vi "APU + 1 Data Replay.vi"() -> ()   [LabVIEW 2013]
uses:
  IP Source/APU/Settings.ctl
  IP Source/APU/Output.ctl
  IP Source/APU/Input.ctl
  IP Source/Analog Replay/Settings.ctl
  IP Source/Analog Replay/Input.ctl
  IP Source/Analog Replay/Load Input.ctl
  IP Source/Version Token.ctl
  IP Source/APU/Shared Settings.ctl
  <vilib>/Platform/TimedLoop/XDataNode/timing_clust.ctl
  <vilib>/Platform/TimedLoop/XDataNode/nitl_modes.ctl
  <vilib>/Platform/TimedLoop/XDataNode/wakeup.ctl
  <vilib>/rvi/DataTransferAndStorage/Container/Common/niFpgaContainerGetUniqueNameForEmu.vi
  <vilib>/rvi/DataTransferAndStorage/Container/Common/niFpgaContainerSetEmuInfo.vi
  <vilib>/rvi/eio/common/nirviEmuReportErrorAndStop.vi
  <vilib>/rvi/Emulation/niFpgaSctlEmulationGetInTimedLoop.vi
  <vilib>/rvi/Emulation/niFpgaEmulationReportErrorSimple.vi
  <vilib>/rvi/Emulation/niFpgaGetClockAttributes.vi
  <vilib>/rvi/Emulation/niFpgaCriticalErrorInLSC.vi
  <vilib>/rvi/eio/common/nirviEmuTemplateMethod_errors.vi
  <vilib>/Platform/TimedLoop/XDataNode/XDataNode.xnode
  <vilib>/rvi/LocalResourceManager/LocalResourceManager.xnode
  <vilib>/eio/EIONode/EIONode.xnode
  <vilib>/Platform/TimedLoop/XDataNode/XDNodeRunTimeDep.lvlib
  IP Source/APU/APU.lvlib
  IP Source/Analog Replay/Analog Replay.lvlib
  IP Source/Engine Simulation Toolkit.lvlib
panel:
  in  "go.my apu":bool
  in  "shared settings.my apu":T1 {"cycle start" format="%#.15g"}
  in  "est.version":T2
  in  "load input.my replay":T3={"Data"=[0, 0, 0, 0, 0, 0, 0, 0, 0, 0, 0, 0, 0, 0, 0, 0], "LoadOffset"=0, "Done"=FALSE}
  in  "input.my replay":T4 caption="input"
  in  "settings.my replay":T5 caption="settings"
  in  "input.my apu":T6={"desired speed"=0.0, "reset"=TRUE} caption="input"
  out "output.my apu":T7 caption="output"
  in  "settings.my apu":T8 caption="settings"
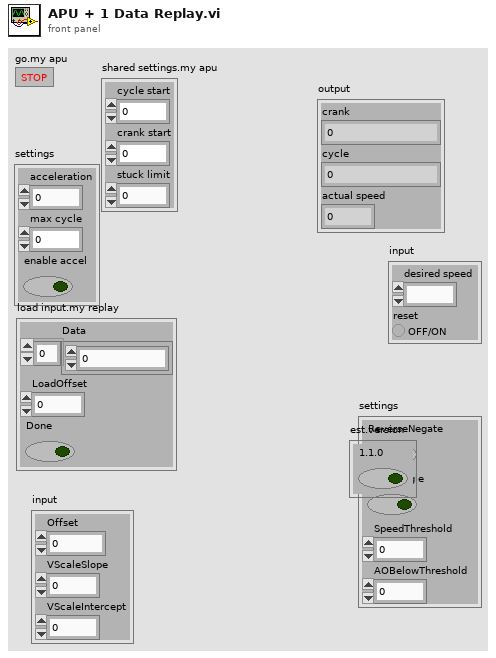
[diagram p1: front panel]
types:
  T1 = typedef "Engine Simulation Toolkit.lvlib/APU.lvlib/Shared Settings.ctl" = cluster{"cycle start":fxp<+,2,2>, "crank start":u16, "stuck limit":fxp<+,18,18>}
  T2 = typedef "Engine Simulation Toolkit.lvlib/Version Token.ctl" = cluster{"1.1.0":bool}
  T3 = typedef "Engine Simulation Toolkit.lvlib/Analog Replay.lvlib/Load Input.ctl" = cluster{"Data":i16[], "LoadOffset":u16, "Done":bool}
  T4 = typedef "Engine Simulation Toolkit.lvlib/Analog Replay.lvlib/Input.ctl" = cluster{"Offset":i16, "VScaleSlope":fxp<+,18,6>, "VScaleIntercept":fxp<+/-,18,3>}
  T5 = typedef "Engine Simulation Toolkit.lvlib/Analog Replay.lvlib/Settings.ctl" = cluster{"ReverseNegate":bool, "CycleAngle":bool, "SpeedThreshold":fxp<+/-,23,2>, "AOBelowThreshold":i16}
  T6 = typedef "Engine Simulation Toolkit.lvlib/APU.lvlib/Input.ctl" = cluster{"desired speed":fxp<+/-,23,2>, "reset":bool}
  T7 = typedef "Engine Simulation Toolkit.lvlib/APU.lvlib/Output.ctl" = cluster{"crank":u16, "cycle":u16, "actual speed":fxp<+/-,23,2>}
  T8 = typedef "Engine Simulation Toolkit.lvlib/APU.lvlib/Settings.ctl" = cluster{"acceleration":fxp<+,18,-20>, "max cycle":fxp<+,2,2>, "enable accel":bool}
  T9 = typedef "XDNodeRunTimeDep.lvlib/timing_clust.ctl" = cluster{"Expected End [f-1]":u64, "Actual End [f-1]":u64, "Finished Late? [f-1]":bool, "Expected End [i-1]":u64, "Actual End [i-1]":u64, "Finished Late? [i-1]":bool, "Expected Start [i]":u64, "Actual Start [i]":u64, "Expected Start [f]":u64, "Actual Start [f]":u64, "Source Name":string, "Structure Name":string, "Period":i64, "Deadline":i64, "Offset":i64, "Start":i64, "Priority":i32, "Timeout":i32, "Mode":T10, "Wakeup Reason":T11, "Error":errorcluster, "Source Type":string, "Secondary Source Type":string, "Global End Time":u64, "Global Start Time":u64, "Frame Duration":u64, "Iteration Duration":u64, "Assigned CPU":i32, "I/O Scan Engine Mode":u32}
  T10 = typedef "XDNodeRunTimeDep.lvlib/nitl_modes.ctl" = enum32{"No Change", "Process missed periods, maintain original phase", "Discard missed periods, maintain original phase", "Process missed periods, ignore original phase", "Discard missed periods, ignore original phase"}
  T11 = typedef "XDNodeRunTimeDep.lvlib/wakeup.ctl" = enum32{"Normal", "Aborted", "Asynchronous wakeup", "Timing source error", "Timed loop error", "Timeout"}
  T12 = typedef "Engine Simulation Toolkit.lvlib/APU.lvlib/Register Bus.ctl" = cluster{"Speed":refnum<k21>, "Crank Angle":refnum<k21>, "Cycle Angle":refnum<k21>, "Crank Count":refnum<k21>, "Cycle Count":refnum<k21>, "1.25 MHz Counter":refnum<k21>, "shared settings":T1}
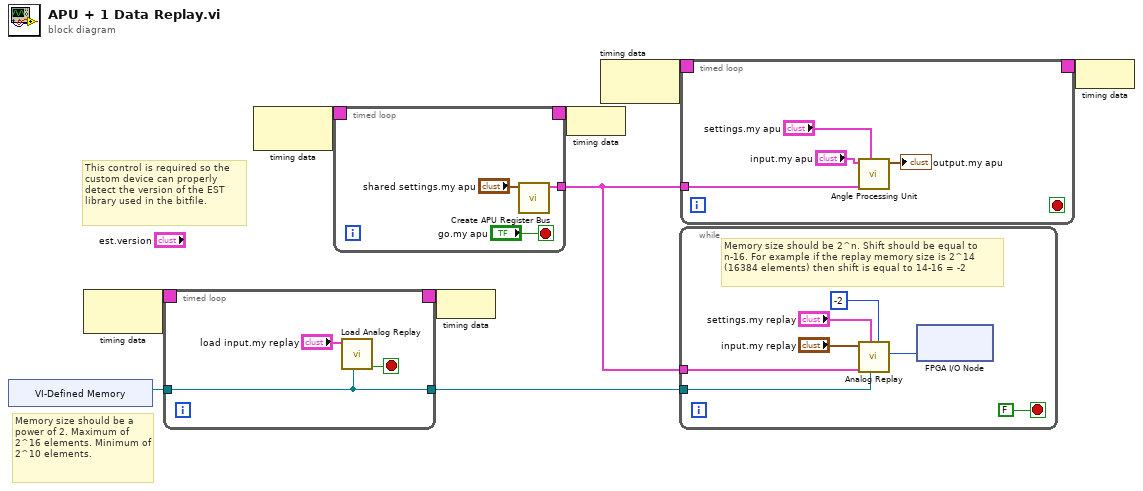
[diagram p0: block diagram]
diagram:
  # "This control is required so the custom device can properly detect the version of the EST library used in the bitfile."
  # "Memory size should be a power of 2. Maximum of 2^16 elements. Minimum of 2^10 elements."
  n1 = xnode "VI-Defined Memory"() -> ("Memory Out"=w7:refnum<k21>)
  n2 = node-c288() -> (w4:T9)  [unwired: 1 in]
  n3 = timed-loop {
    tunnel: w7 -> [w11]
    tunnel: [w11] -> w6
    timing: w4 -> [_]
    timing-out: [_] -> w3
    stop <- w12 stop-if-true
    n4 = call "Load Analog Replay.vi"("memory"=w11, "load input.<user name>"="load input.my replay") -> ("done"=w12:bool)  [unwired: 9 in]
  }
  n5 = node-c288() -> (w2:T9)  [unwired: 1 in]
  n6 = timed-loop {
    timing: w2 -> [_]
    timing-out: [_] -> w1
    tunnel: [w17] -> w5
    stop <- "go.my apu" stop-if-true
    n7 = call "Create APU Register Bus.vi"("shared settings.<user name>"="shared settings.my apu") -> ("register bus"=w17:T12)  [unwired: 10 in]
  }
  n8 = node-c288(w3) -> ()
  n9 = node-c288(w1) -> ()
  n10 = node-c288() -> (w9:T9)  [unwired: 1 in]
  n11 = while {
    tunnel: w6 -> [w26]
    tunnel: w5 -> [w23]
    stop <- FALSE stop-if-true
    # "Memory size should be 2^n. Shift should be equal to n-16. For example if the replay memory size is 2^14 (16384 elements) then shift is equal to 14-16 = -2"
    n12 = call "Analog Replay.vi"("shift"=i8 -2, "memory"=w26, "settings.<user name>"="settings.my replay", "register bus"=w23, "input.<user name>"="input.my replay") -> ("analog value"=w21:i16)  [unwired: 6 in]
    n13 = xnode "FPGA I/O Node"("AO0"=w21) -> ()  [unwired: 1 in, 1 out]
  }
  n14 = timed-loop {
    timing: w9 -> [_]
    timing-out: [_] -> w8
    tunnel: w5 -> [w27]
    stop <- _ stop-if-true
    n15 = call "Angle Processing Unit.vi"("settings.<user name>"="settings.my apu", "register bus"=w27, "input.<user name>"="input.my apu") -> ("output.<user name>"=→"output.my apu":T7)  [unwired: 8 in]
  }
  n16 = node-c288(w8) -> ()
